vi "5.3 - Waypoint Min Max.vi"(0 "6.2 MDF to Neo-Cortex":T1[](array[typedef]) {"X (waypoint)" format="%#_8g"; "Y  (waypoint)" format="%#_8g"}) -> (1 "Y Dimension (Row)":ext, 2 "X Dimension (Column)":ext)   [LabVIEW 2010]
uses:
  6-OCU Neurons/MDF XY.ctl
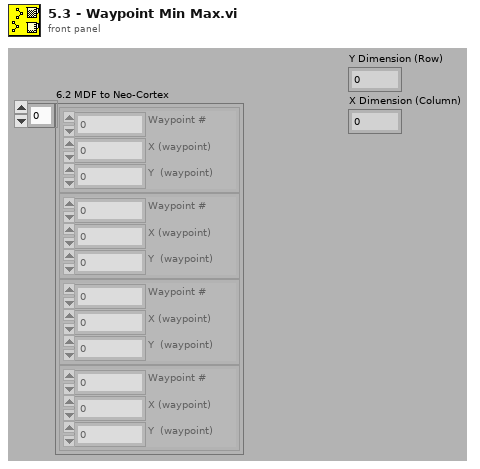
[diagram p1: front panel]
types:
  T1 = typedef "MDF XY.ctl" = cluster{"Waypoint #":dbl, "X (waypoint)":ext, "Y  (waypoint)":ext}
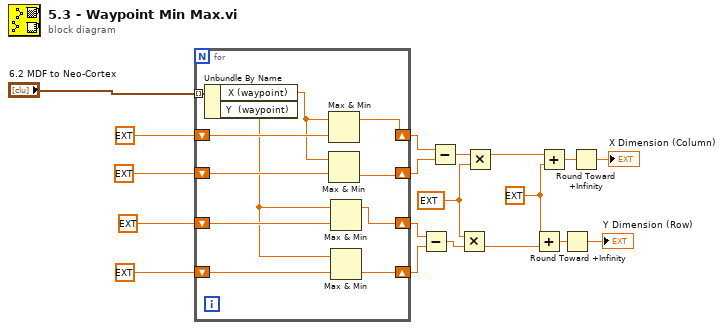
[diagram p0: block diagram]
diagram:
  w3 = ext 3.28 ("x")
  w6 = ext 50.0 ("x")
  n1 = for {
    tunnel: "6.2 MDF to Neo-Cortex" -> [w30] mode=indexing
    shift-right: [w28] -> w14
    shift-left: ext 0.0 -> [w29]
    shift-right: [w26] -> w12
    shift-left: ext 0.0 -> [w27]
    shift-right: [w23] -> w13
    shift-left: ext 0.0 -> [w24]
    shift-right: [w20] -> w11
    shift-left: ext 0.0 -> [w21]
    n2 = Unbundle By Name(w30) -> ("X (waypoint)"=w25:ext, "Y  (waypoint)"=w22:ext)
    n3 = Max & Min(x=w25, y=w29) -> (max(x,y)=w28:ext)  [unwired: 1 out]
    n4 = Max & Min(x=w25, y=w24) -> (min(x,y)=w23:ext)  [unwired: 1 out]
    n5 = Max & Min(x=w22, y=w27) -> (max(x,y)=w26:ext)  [unwired: 1 out]
    n6 = Max & Min(x=w22, y=w21) -> (min(x,y)=w20:ext)  [unwired: 1 out]
  }
  n7 = Subtract(x=w12, y=w11) -> (x-y=w7:ext)
  n8 = Subtract(x=w14, y=w13) -> (x-y=w10:ext)
  n9 = Multiply(x=w3, y=w7) -> (x*y=w4:ext)
  n10 = Multiply(x=w10, y=w3) -> (x*y=w5:ext)
  n11 = Add(x=w6, y=w4) -> (x+y=w8:ext)
  n12 = Add(x=w5, y=w6) -> (x+y=w9:ext)
  n13 = Round Toward +Infinity(x=w8) -> (ceil(x): smallest int >= x=→"Y Dimension (Row)":ext)
  n14 = Round Toward +Infinity(x=w9) -> (ceil(x): smallest int >= x=→"X Dimension (Column)":ext)
